vi "Add Routing and Faulting Custom Device.vi"(8 "error in (no error)":errorcluster, 11 "Target in":refnum<k24>) -> (0 "error out":errorcluster, 1 "Aliases Section Ref":T1 format="%.0x", 2 "RaF CD Ref":T1 format="%.0x", 3 "Target out":refnum<k24>, 4 "Routes Section Ref":T1 format="%.0x")   [LabVIEW 2017, in "SLSC Switch Scripting.lvlib"]
uses:
  SLSC Switch Scripting.lvlib
  NationalInstruments.VeriStand.SystemDefinitionAPI
  <vilib>/NI Veristand/Custom Device API/Custom Device Item Ref.ctl
  SLSC Scripting Constants.vi
  <vilib>/NI VeriStand/Custom Device API/Custom Device API.lvlib
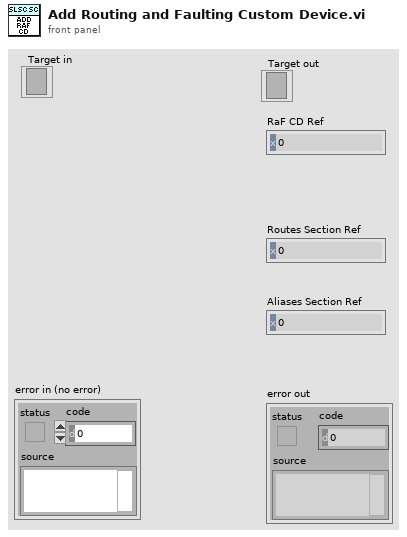
[diagram p1: front panel]
types:
  T1 = typedef "Custom Device API.lvlib/Custom Device Item Ref.ctl" = u64
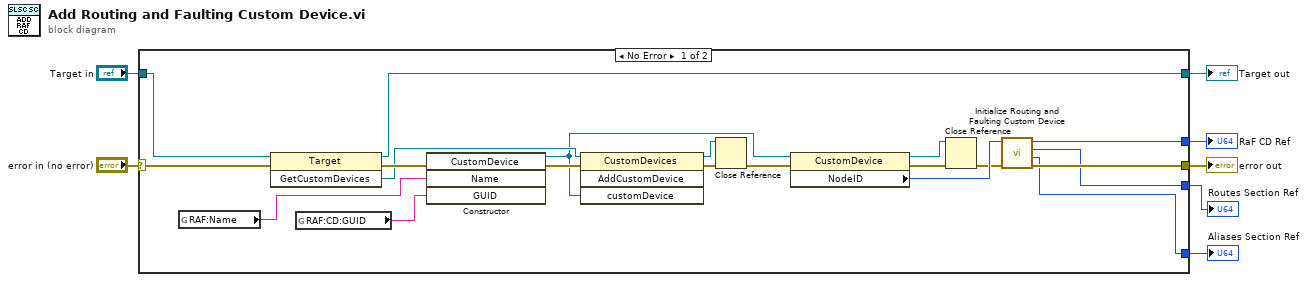
[diagram p0: block diagram]
diagram:
  n1 = case shown="No Error" "error in (no error)" {
    selector: "error in (no error)" -> [w27 w29]
    tunnel: [w15 w29] -> w7
    tunnel: "Target in" -> [w26 w28]
    tunnel: [w22 w28] -> w4
    tunnel: [w14 _] -> w3
    tunnel: [w13 _] -> w2
    tunnel: [w11 _] -> w1
    frame No Error {
      n2 = global read "SLSC Scripting Constants.vi" "RAF:Name"() -> (w12:string)
      n3 = invoke class="Target" method="GetCustomDevices"(reference=w26, error in=w27) -> (reference out=w22:refnum<k24>, error out=w25:errorcluster, "GetCustomDevices"=w24:refnum<k24>)  [unwired: 1 in]
      n4 = global read "SLSC Scripting Constants.vi" "RAF:CD:GUID"() -> (w17:string)
      n5 = constructor class="CustomDevice"(error in=w25, "Name"=w12, "GUID"=w17) -> (reference out=w19:refnum<k24>, error out=w23:errorcluster)  [unwired: 2 in, 3 out]
      n6 = invoke class="CustomDevices" method="AddCustomDevice"(reference=w24, error in=w23, "customDevice"=w19) -> (reference out=w21:refnum<k24>, error out=w20:errorcluster)  [unwired: 1 in, 2 out]
      n7 = Close Reference(reference=w21, error in (no error)=w20) -> (error out=w18:errorcluster)
      n8 = property class="CustomDevice"(reference=w19, error in=w18) -> (reference out=w10:refnum<k24>, error out=w9:errorcluster, "NodeID"=w16:u64)
      n9 = Close Reference(reference=w10, error in (no error)=w9) -> (error out=w8:errorcluster)
      n10 = call "Initialize Routing and Faulting Custom Device.vi"("error in (no error)"=w8, "RaF CD Ref in"=w16) -> ("error out"=w15:errorcluster, "Aliases Section Ref"=w13:T1, "Routes Section Ref"=w14:T1, "RaF CD Ref out"=w11:T1)  [unwired: 6 in]
    }
    frame Error {
    }
  }
  "Target out" <- w4
  "error out" <- w7
  "RaF CD Ref" <- w1
  "Routes Section Ref" <- w3
  "Aliases Section Ref" <- w2
